vi "Library Folder.vi"() -> (3 "Library Folder":path)   [LabVIEW 2020, in "HAL.lvlib" / "HAL Manager.lvclass"]
uses:
  HAL Manager.lvclass
  <vilib>/Utility/LVLibp/NI_PackedLibraryUtility.lvlib
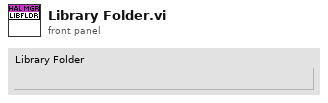
[diagram p1: front panel]
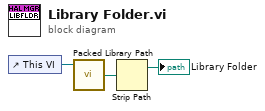
[diagram p0: block diagram]
diagram:
  n1 = control-ref of="This VI"() -> (w3:refnum<vi>)
  n2 = call <vilib>:"Packed Library Path.vi"("vi reference"=w3) -> ("packed library path"=w2:path)  [unwired: 2 in, 2 out]
  n3 = Strip Path(path=w2) -> (stripped path=→"Library Folder":path)  [unwired: 1 out]
